vi "Parse Installed Files.vi"(8 "Error In":errorcluster, 10 "Files Installed":path[](array[path]), 11 "Dependecy Config in":T1) -> (0 "Error Out":errorcluster, 2 "Config Found?":bool, 3 "Dependecy Config out":T1)   [LabVIEW 2011, in "LVH-Toolbox.lvlib" / "Installer Tools.lvlib"]
uses:
  Installer Tools.lvlib
  Type Defs/Dependency Config.ctl
  Type Defs/Dependecy.ctl
  Common/Private/Web/Type Defs/Download Task.ctl
  Common/LVH-Common.lvlib
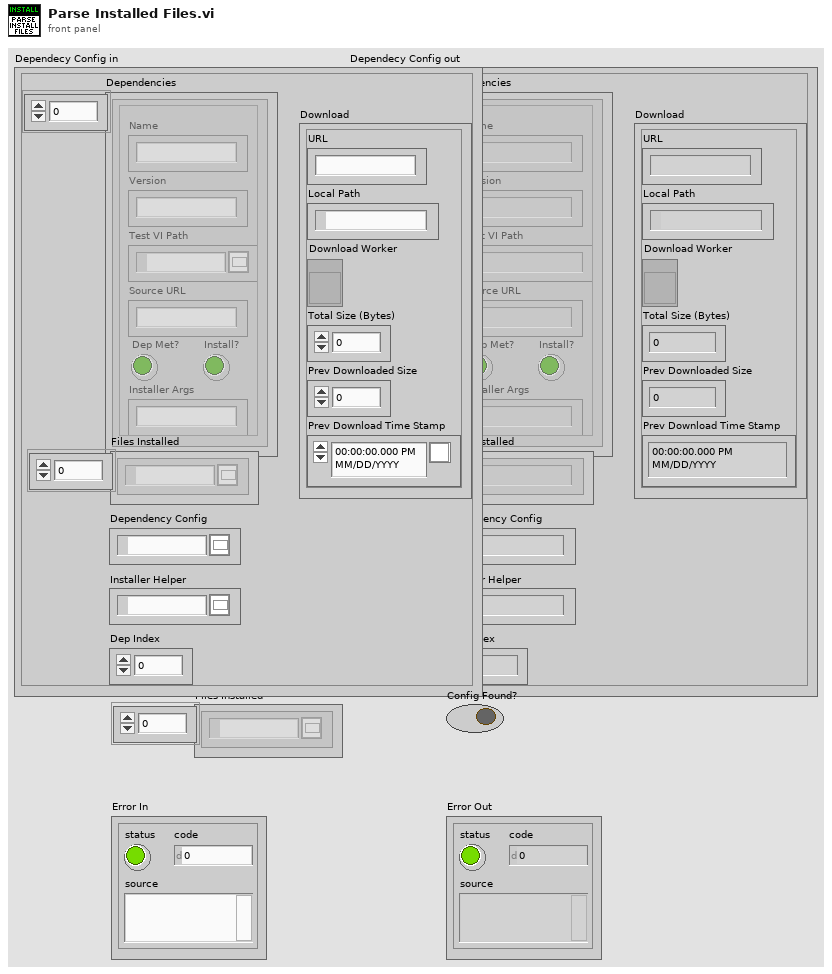
[diagram p1: front panel]
types:
  T1 = typedef "LVH-Toolbox.lvlib/Installer Tools.lvlib/Dependency Config.ctl" = cluster{"Dependencies":T2[], "Files Installed":path[], "Dependency Config":path, "Installer Helper":path, "Dep Index":i32, "Download":T3}
  T2 = typedef "LVH-Toolbox.lvlib/Installer Tools.lvlib/Dependecy.ctl" = cluster{"Name":string, "Version":string, "Test VI Path":path, "Source URL":string, "Dep Met?":bool, "Install?":bool, "Installer Args":string}
  T3 = typedef "LVH-Toolbox.lvlib/LVH-Common.lvlib/Download Task.ctl" = cluster{"URL":string, "Local Path":path, "Download Worker":refnum<vi>, "Total Size (Bytes)":u64, "Prev Downloaded Size":u64, "Prev Download Time Stamp":timestamp}
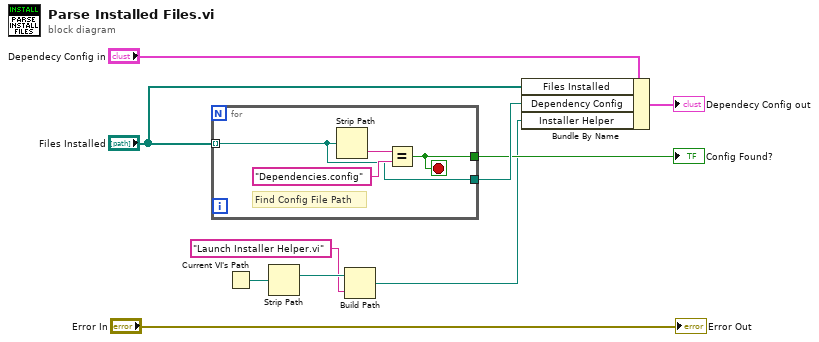
[diagram p0: block diagram]
diagram:
  n1 = for {
    tunnel: "Files Installed" -> [w11] mode=indexing
    tunnel: [w12] -> w6
    tunnel: [w11] -> w9
    stop <- w12 stop-if-true
    # "Find Config File Path"
    n2 = Strip Path(path=w11) -> (name=w14:string)  [unwired: 1 out]
    n3 = Equal?(x=w14, y="Dependencies.config") -> (x = y?=w12:bool)
  }
  "Config Found?" <- w6
  n4 = Current VI's Path() -> (path=w3:path)
  n5 = Strip Path(path=w3) -> (stripped path=w4:path)  [unwired: 1 out]
  n6 = Build Path(base path=w4, name or relative path="Launch Installer Helper.vi") -> (appended path=w2:path)
  n7 = Bundle By Name(cluster="Dependecy Config in", "Files Installed"="Files Installed", "Dependency Config"=w9, "Installer Helper"=w2) -> (→"Dependecy Config out":T1)
  "Error Out" <- "Error In"
